vi "GPS Path History.vi"(9 "Initial Latitiude":dbl, 10 "Initial Longitude":dbl, 11 "VISA resource name":refnum<visa-resource-name>) -> (1 "Latitude Dist":dbl, 2 "Longitude Dist":dbl)   [LabVIEW 2009]
uses:
  GPS Read VISA Instance.vi
panel:
  out "GPS X-Y Plot":cluster{dbl, dbl}[](graph)
  out "GPS Relative Path History (XY)":cluster{dbl, dbl}[](array[cluster])
  in  "stop":bool
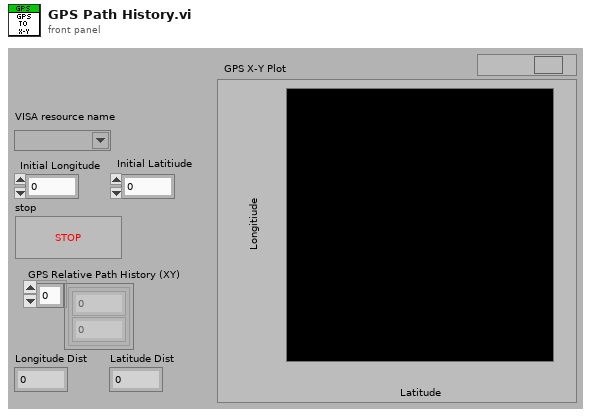
[diagram p1: front panel]
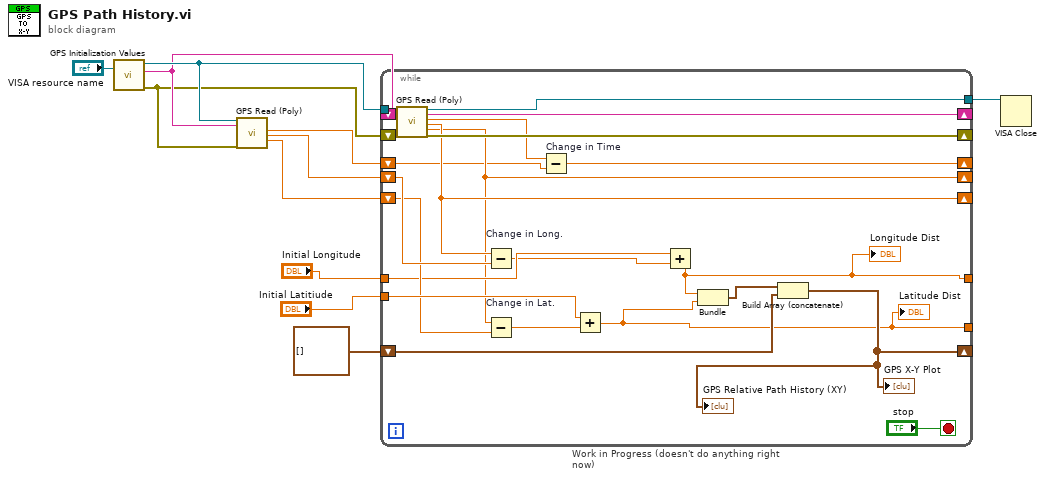
[diagram p0: block diagram]
diagram:
  n1 = call "GPS Initialization Values.vi"("VISA resource name"="VISA resource name") -> ("error In"=w7:errorcluster, "Buffer In"=w8:string, "VISA resource name In"=w9:refnum<visa-resource-name>)  [unwired: 8 in]
  n2 = call-poly "GPS Read (Poly).vi"("VISA In"=w9, "Buffer In"=w8, "Error In"=w7) -> ("Time"=w6:dbl, "Longitude"=w2:dbl, "Latitude"=w1:dbl)  [unwired: 10 in, 4 out]
  n3 = while "Work in Progress (doesn't do anything right now)" {
    tunnel: "Initial Latitiude" -> [w34]
    tunnel: w9 -> [w31]
    shift-right: [w28] -> _
    shift-left: w8 -> [w29]
    tunnel: [w27] -> w10
    shift-right: [w26] -> _
    shift-left: w7 -> [w30]
    shift-right: [w21] -> _
    shift-left: w2 -> [w25]
    shift-right: [w23] -> _
    shift-left: w1 -> [w24]
    tunnel: "Initial Longitude" -> [w22]
    shift-right: [w19] -> _
    shift-left: w6 -> [w18]
    shift-right: [w15] -> _
    shift-left: cluster{dbl, dbl}[] [] -> [w16]
    tunnel: [w14] -> _
    tunnel: [w13] -> _
    stop <- "stop" stop-if-true
    n4 = call-poly "GPS Read (Poly).vi"("VISA In"=w31, "Buffer In"=w29, "Error In"=w30) -> ("VISA Out"=w27:refnum<visa-resource-name>, "Buffer Out"=w28:string, "Time"=w20:dbl, "Longitude"=w23:dbl, "Latitude"=w21:dbl, "Error Out"=w26:errorcluster)  [unwired: 10 in, 1 out]
    n5 = Subtract "Change in Long."(x=w23, y=w25) -> (x-y=w12:dbl)
    n6 = Subtract "Change in Lat."(x=w21, y=w24) -> (x-y=w33:dbl)
    n7 = Subtract "Change in Time"(x=w20, y=w18) -> (x-y=w19:dbl)
    n8 = Add(x=w34, y=w33) -> (x+y=w13:dbl)
    "Latitude Dist" <- w13
    n9 = Add(x=w22, y=w12) -> (x+y=w14:dbl)
    "Longitude Dist" <- w14
    n10 = Bundle(w14, w13) -> (w17:cluster{dbl, dbl})  [unwired: 1 in]
    n11 = Build Array (concatenate)(w17, w16) -> (w15:cluster{dbl, dbl}[])
    "GPS X-Y Plot" <- w15
    "GPS Relative Path History (XY)" <- w15
  }
  n12 = VISA Close(VISA resource name=w10) -> ()  [unwired: 1 in, 1 out]
